vi "Release-queues.vi"(8 "error in (no error)":errorcluster, 11 "Buffers in":refnum<class "CV-Buffers.lvclass">) -> (0 "error out":errorcluster, 3 "Buffers out":refnum<class "CV-Buffers.lvclass">)   [LabVIEW 2013, in "CameraVision.lvlib" / "CV-Buffers.lvclass"]
uses:
  CV-Buffers.lvclass
  CV-Buffers.lvclass/CV-Buffers.ctl
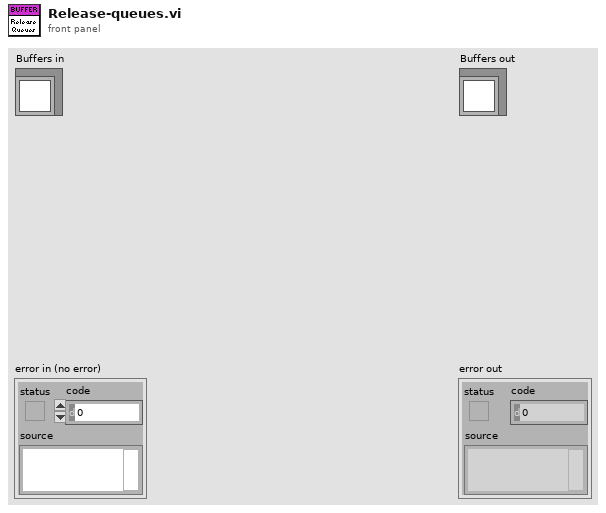
[diagram p1: front panel]
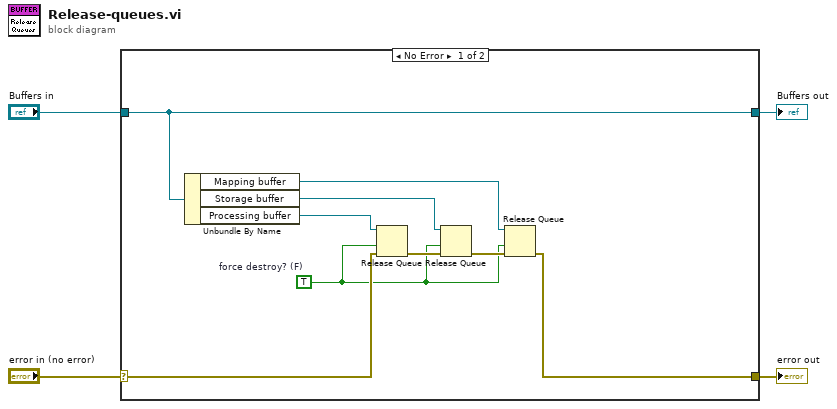
[diagram p0: block diagram]
diagram:
  n1 = case shown="No Error" "error in (no error)" {
    selector: "error in (no error)" -> [w9 w15]
    tunnel: [w12 w15] -> w3
    tunnel: [w13 w14] -> w1
    tunnel: "Buffers in" -> [w13 w14]
    frame No Error {
      w5 = TRUE  # force destroy? (F)
      n2 = Unbundle By Name(w13) -> ("Mapping buffer"=w8:refnum<queue>, "Storage buffer"=w7:refnum<queue>, "Processing buffer"=w6:refnum<queue>)
      n3 = Release Queue(queue=w6, force destroy? (F)=w5, error in (no error)=w9) -> (error out=w10:errorcluster)  [unwired: 2 out]
      n4 = Release Queue(queue=w7, force destroy? (F)=w5, error in (no error)=w10) -> (error out=w11:errorcluster)  [unwired: 2 out]
      n5 = Release Queue(queue=w8, force destroy? (F)=w5, error in (no error)=w11) -> (error out=w12:errorcluster)  [unwired: 2 out]
    }
    frame Error {
    }
  }
  "error out" <- w3
  "Buffers out" <- w1
